vi "Check Variant Type.vi"(8 "error in (no error)":errorcluster, 10 "Variant In":variant, 11 "Numeric Field in":refnum<class "Numeric Field.lvclass">) -> (0 "error out":errorcluster, 2 "Variant Out":variant, 3 "Numeric Field out":refnum<class "Numeric Field.lvclass">)   [LabVIEW 2020]
uses:
  Numeric Field.lvclass
panel:
  # "For override: Check that variant type is compatible with field control object"
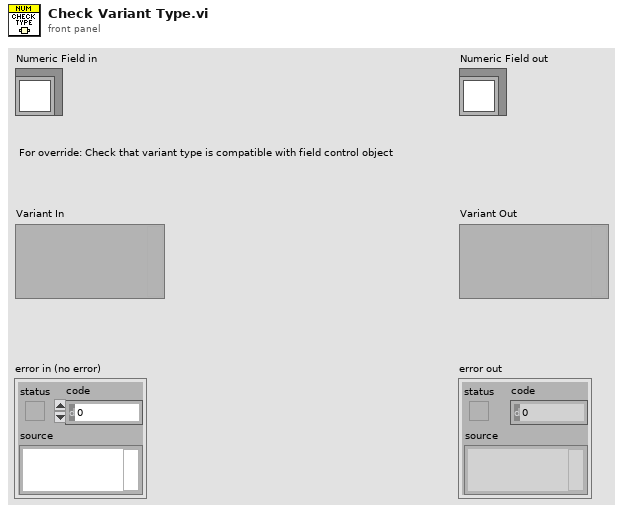
[diagram p1: front panel]
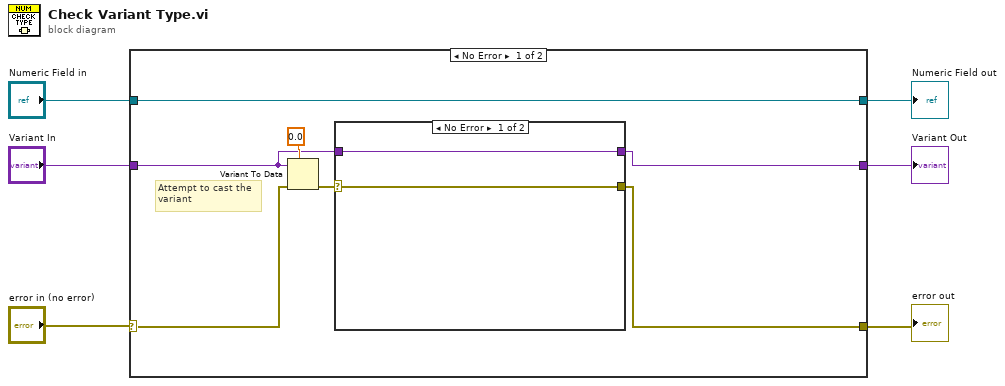
[diagram p0: block diagram]
diagram:
  n1 = case shown="No Error" "error in (no error)" {
    selector: "error in (no error)" -> [w8 w18]
    tunnel: [w7 w18] -> w5
    tunnel: "Variant In" -> [w10 w20]
    tunnel: [w9 w20] -> w3
    tunnel: "Numeric Field in" -> [w13 w19]
    tunnel: [w13 w19] -> w1
    frame No Error {
      # "Attempt to cast the\nvariant"
      n2 = Variant To Data(error in=w8, type=0.0, Variant=w10) -> (error out=w11:errorcluster)  [unwired: 1 out]
      n3 = case shown="No Error" w11 {
        selector: w11 -> [w14 w16]
        tunnel: w10 -> [w15 w17]
        tunnel: [w15 w17] -> w9
        tunnel: [w14 w16] -> w7
        frame No Error {
        }
        frame Error {
          # "todo: add error handling, codes, etc"
        }
      }
    }
    frame Error {
    }
  }
  "error out" <- w5
  "Numeric Field out" <- w1
  "Variant Out" <- w3
